vi "Impulse Response (V1.00).vi"(0 "wFormDSP Ref IN":refnum<class "GSwFormDSP.lvclass">, 5 "error in (no error)":errorcluster, 6 "ReInit All to Default?":bool, 7 "Application Name":string="GenUtil", 9 "State Queue":T1[](array[typedef])=["SC >>> Initialize"]) -> (19 "error out":errorcluster)   [LabVIEW 2020, in "SigMath.lvclass"]
uses:
  SigMath.lvclass
  API/Generic Utilities_class/utils/GenUtil State List.ctl
  API/GSwFormDSP_class/GSwFormDSP.lvclass
  <vilib>/Utility/sysdir.llb/System Directory Type.ctl
  API/GSwFormDSP_class/functions/Transfer Function Type.ctl
  C:/Users/fcharett/docsWork/coding/20openSourceSPWB/API/Generic Utilities_class/Generic Utilities.lvclass
  <vilib>/Platform/browser.llb/Open URL in Default Browser (path).vi
  <vilib>/addons/_AddQ/G#Object/G#Object.lvclass
  API/Generic Utilities_class/Generic Utilities.lvclass
  File IO/TEXT_class/TEXT.lvclass
panel:
  in  "Task":enum32{"Monitor", "Settings"}(tab)
  in  "Frequency Intervals [Hz]":u16(ring) items=["No Change", "0.10 Hz", "0.25 Hz", "0.50 Hz", "1.0 Hz", "2.0 Hz", "5.0 Hz", "10 Hz "]
  in  "Impulse Response":waveform(dbl)[](graph)
  out "Spectrum":cluster{dbl[], "Y":dbl[]}[](graph)
  in  "Exit":bool
  in  "Select CSV File":bool
  in  "AppData Folder":bool
  out "State History":string[](array[string])
  out "State Index":i32
  out "Exec Time":dbl
  out "Created New OBJ?":bool
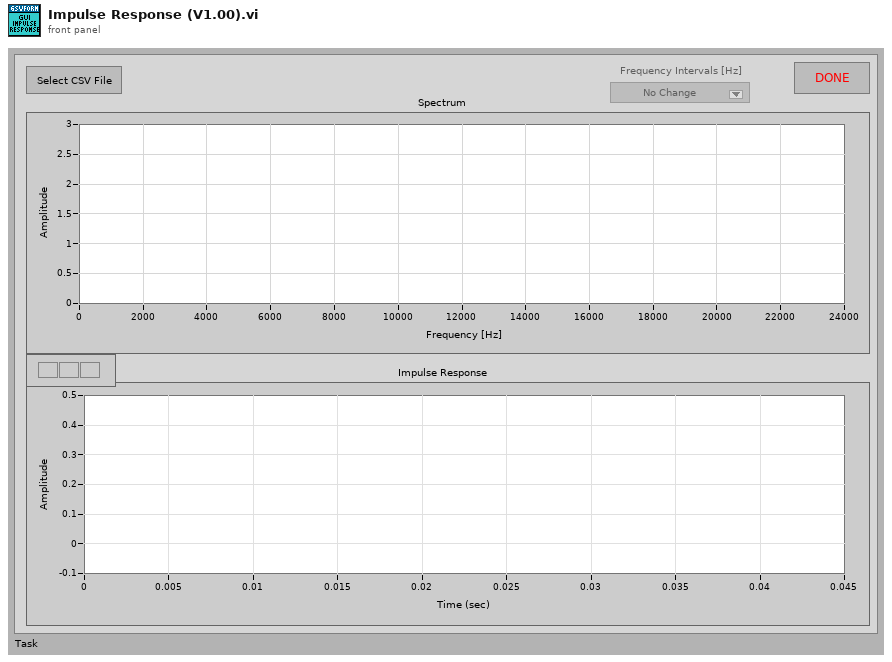
[diagram p1: front panel]
types:
  T1 = typedef "Generic Utilities.lvclass/GenUtil State List.ctl" = string
  T2 = typedef "GSwFormDSP.lvclass/Transfer Function Type.ctl" = enum16{"Magnitude", "Phase (Rad)", "Phase Unwrap (Rad)", "Phase (Degree)", "Phase Unwrap (Degree)", "Coherence"}
  T3 = enum32{"Invalid", "Standard", "Closed", "Hidden", "Minimized", "Maximized"}
  T4 = typedef "System Directory Type.ctl" = i32
  T5 = typedef "SigMath.lvclass/SigMath Data.ctl" = cluster{"New Time Data Obj?":bool, "GSwFormDSP":refnum<class "GSwFormDSP.lvclass">}
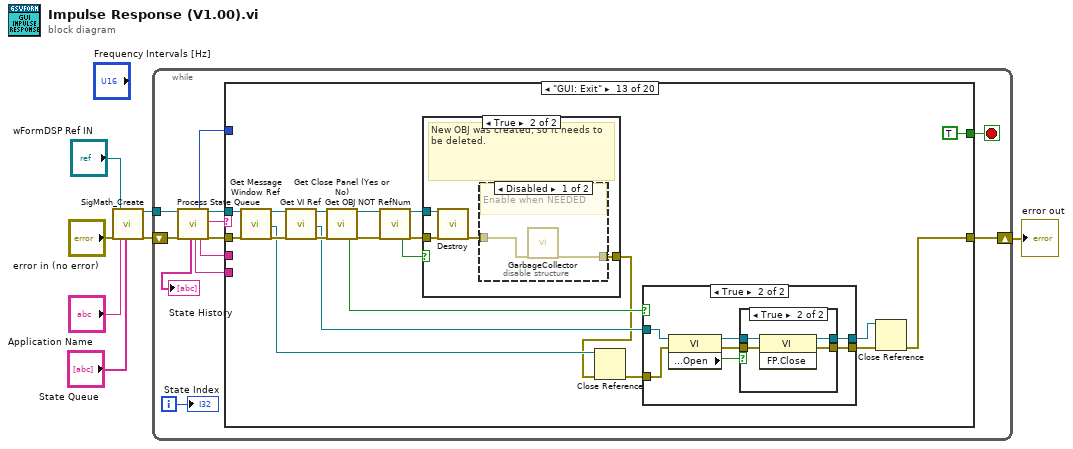
[diagram p0: block diagram]
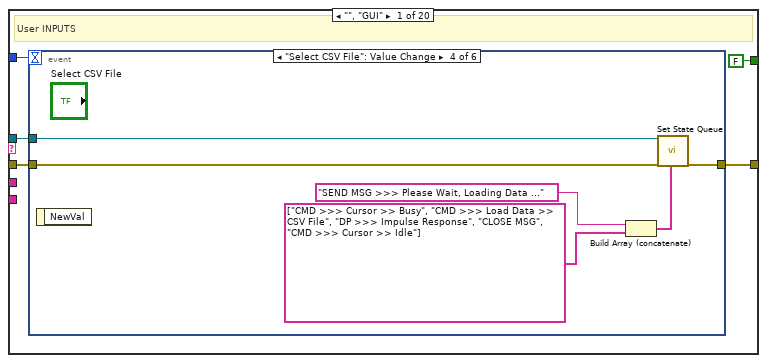
[diagram p2: hidden frame]
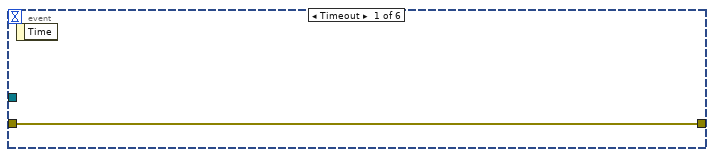
[diagram p3: hidden frame]
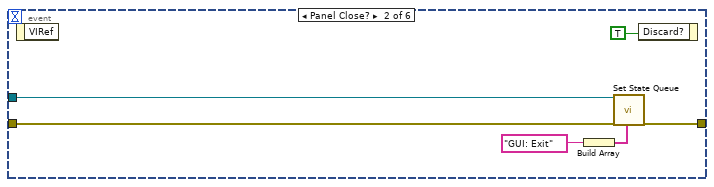
[diagram p4: hidden frame]
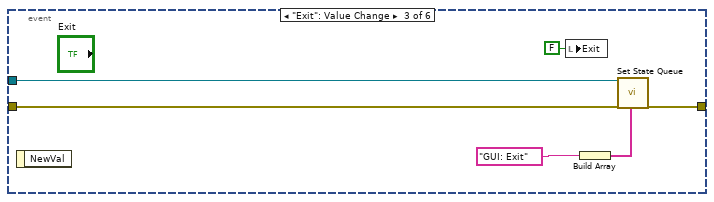
[diagram p5: hidden frame]
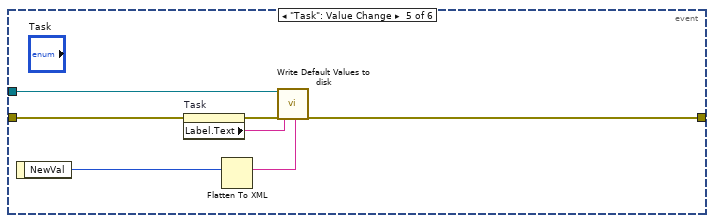
[diagram p6: hidden frame]
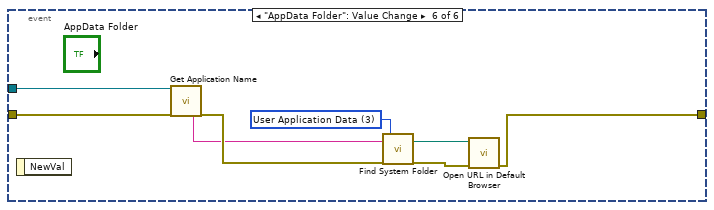
[diagram p7: hidden frame]
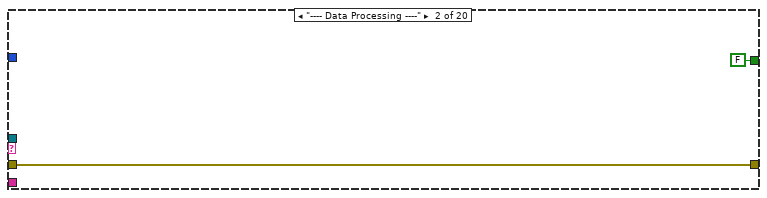
[diagram p8: hidden frame]
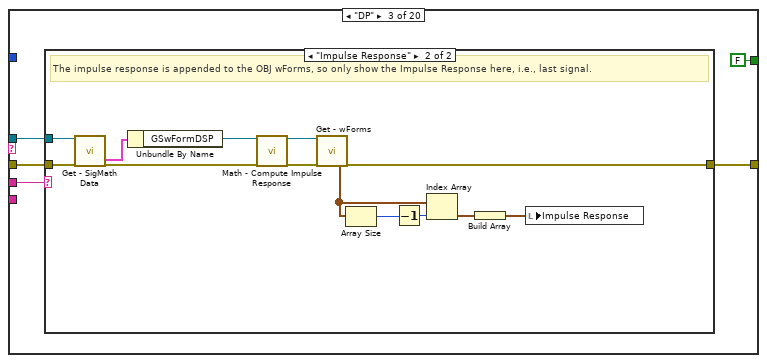
[diagram p9: hidden frame]
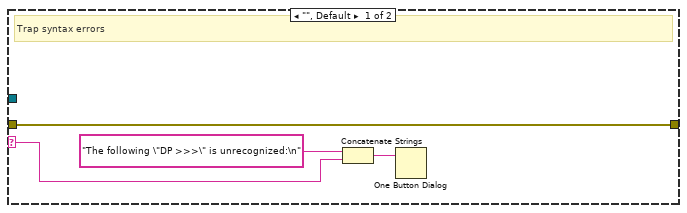
[diagram p10: hidden frame]
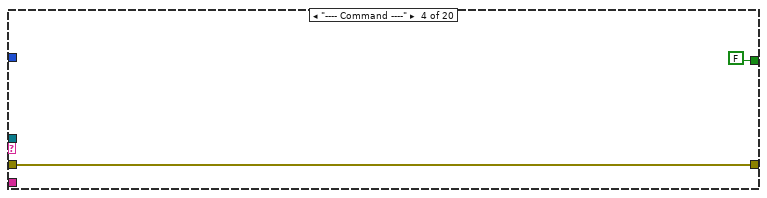
[diagram p11: hidden frame]
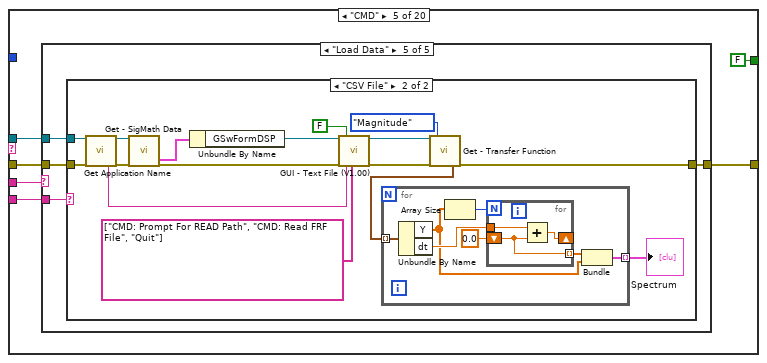
[diagram p12: hidden frame]
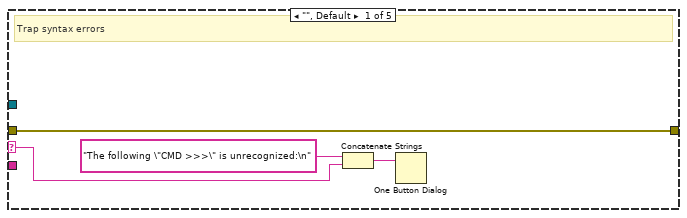
[diagram p13: hidden frame]
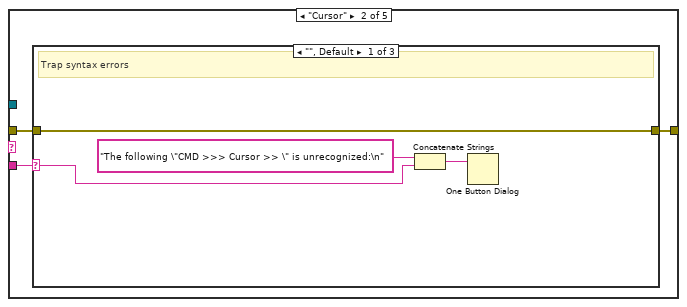
[diagram p14: hidden frame]
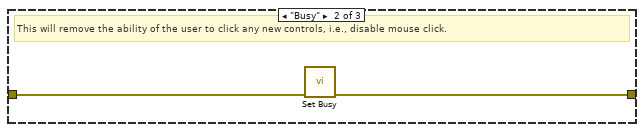
[diagram p15: hidden frame]
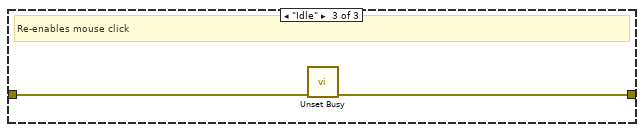
[diagram p16: hidden frame]
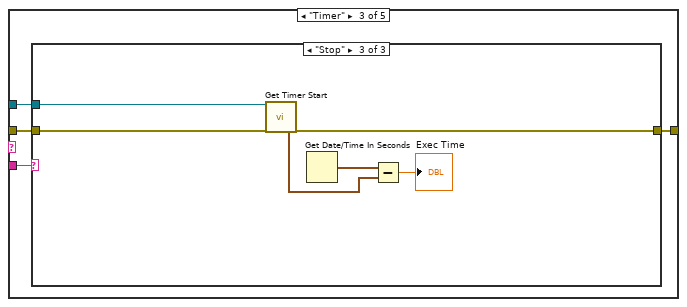
[diagram p17: hidden frame]
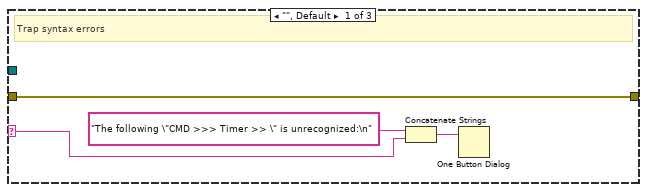
[diagram p18: hidden frame]
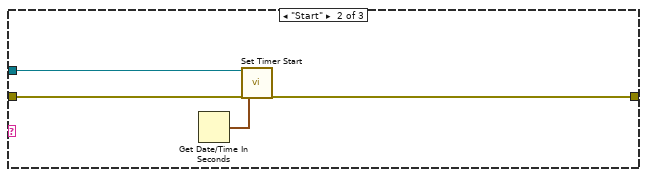
[diagram p19: hidden frame]
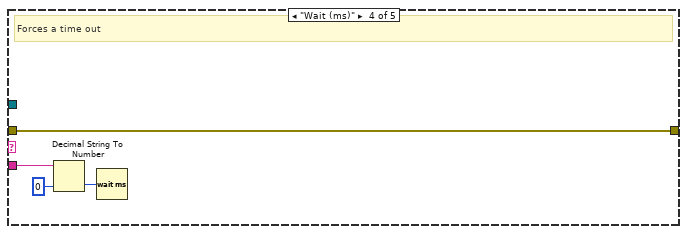
[diagram p20: hidden frame]
diagram:
  n1 = call "SigMath_Create.vi"("error in (no error)"="error in (no error)", "Time Data"="wFormDSP Ref IN", "Application Name"="Application Name", "State Queue"="State Queue") -> ("reference out"=w7:refnum<class "SigMath.lvclass">, "error out"=w6:errorcluster)  [unwired: 14 in]
  n2 = while {
    shift-right: [w11] -> w2
    shift-left: w6 -> [w16]
    tunnel: w7 -> [w17]
    i -> [w18]
    stop <- w19 stop-if-true
    n3 = call "Process State Queue.vi"("reference in"=w17, "error in (no error)"=w16) -> ("State History"=→"State History":string[], "Additional Options"=w8:string, "Timeout"=w15:i32, "State Option"=w10:string, "reference out"=w14:refnum<class "SigMath.lvclass">, "Current State"=w13:string, "error out"=w12:errorcluster)  [unwired: 10 in, 1 out]
    n4 = case shown="\"GUI: Exit\"" w13 {
      selector: w13 -> [_ _ _ _ _ _ _ _ _ _ _ _ _ _ _ _ w348 _ _ _]
      tunnel: w14 -> [w22 _ w61 _ w85 _ w169 _ w180 w214 _ w252 w271 w307 w332 _ _ _ _ w358]
      tunnel: [FALSE FALSE FALSE FALSE FALSE FALSE FALSE FALSE FALSE FALSE FALSE FALSE TRUE FALSE FALSE FALSE FALSE FALSE FALSE TRUE] -> w19
      tunnel: w15 -> [w23 _ _ _ _ _ _ _ _ _ _ _ _ _ _ _ _ _ _ _]
      tunnel: w10 -> [_ _ w64 _ w89 _ w165 _ w181 w211 _ _ _ w316 _ _ _ _ _ _]
      tunnel: w12 -> [w21 w59 w63 w83 w87 w162 w168 w176 w178 w213 w234 w249 w268 w306 w333 w344 w346 w351 w354 w357]
      tunnel: [w20 w59 w62 w83 w88 w162 w167 w176 w179 w212 w234 w241 w267 w304 w329 w344 w346 errorcluster {"status"=FALSE, "code"=0, "source"=""} ("error out") w354 w356] -> w11
      tunnel: w8 -> [_ _ _ _ w86 _ _ _ _ _ _ _ _ _ _ _ _ _ _ _]
      frame "", "GUI" {
        # "User INPUTS"
        n5 = event shown="[3] \"Select CSV File\": Value Change" {
          selector: _ -> [_ _ _ _ _ _]
          dyn-events: _ -> [_ _ _ _ _ _]
          timeout: w23 -> [_ _ _ _ _ _]
          tunnel: w22 -> [_ w30 w36 w42 w49 w57]
          tunnel: w21 -> [w25 w29 w34 w41 w46 w56]
          tunnel: [w25 w28 w35 w43 w44 w51] -> w20
          event Timeout {
            n6 = event-data() -> ()  [unwired: 1 in, 1 out]
          }
          event Panel Close? {
            n7 = event-data() -> ()  [unwired: 1 in, 1 out]
            n8 = Build Array(T1 "GUI: Exit" ("State List")) -> (w27:T1[])
            n9 = call "Set State Queue.vi"("reference in"=w30, "error in (no error)"=w29, "State Queue"=w27) -> ("error out"=w28:errorcluster)  [unwired: 15 in, 1 out]
            n10 = event-data("Discard?"=TRUE) -> ()  [unwired: 1 in, 1 out]
          }
          event "Exit": Value Change {
            n11 = event-data() -> ()  [unwired: 1 in, 1 out]
            n12 = local write "Exit"(FALSE ("Exit")) -> ()
            n13 = Build Array(T1 "GUI: Exit" ("State List")) -> (w33:T1[])
            n14 = call "Set State Queue.vi"("reference in"=w36, "error in (no error)"=w34, "State Queue"=w33) -> ("error out"=w35:errorcluster)  [unwired: 15 in, 1 out]
          }
          event "Select CSV File": Value Change {
            n15 = event-data() -> ()  [unwired: 1 in, 1 out]
            n16 = Build Array (concatenate)("SEND MSG >>> Please Wait, Loading Data ..." ("String"), T1[] ["CMD >>> Cursor >> Busy", "CMD >>> Load Data >> CSV File", "DP >>> Impulse Response", "CLOSE MSG", "CMD >>> Cursor >> Idle"] ("State Queue OUT")) -> (w38:T1[])
            n17 = call "Set State Queue.vi"("reference in"=w42, "error in (no error)"=w41, "State Queue"=w38) -> ("error out"=w43:errorcluster)  [unwired: 15 in, 1 out]
          }
          event "Task": Value Change {
            n18 = event-data() -> ("NewVal"=w50:enum32{"Monitor", "Settings"})  [unwired: 1 in]
            n19 = property on="Task" class="TabCtl (strict)"(error in=w46) -> (error out=w45:errorcluster, "Label.Text"=w48:string)  [unwired: 1 in, 1 out]
            n20 = Flatten To XML(6:w50) -> (2:w47:string)
            n21 = call-dynamic "Write Default Values to disk.vi"("reference in"=w49, "error in (no error)"=w45, "Control Label"=w48, "Value (XML String)"=w47) -> ("error out"=w44:errorcluster)  [unwired: 14 in, 1 out]
          }
          event "AppData Folder": Value Change {
            w58 = T4 3 items=["User Home"=0, "User Desktop"=1, "User Documents"=2, "User Application Data"=3, "User Preferences"=4, "User Temporary"=5, "Public Documents"=6, "Public Application Data"=7, "Public Preferences"=8, "Public Cache"=13, "System Core Libraries"=9, "System Installed Libraries"=10, "Application Files"=11, "Boot Volume Root"=12] ("system directory type")
            n22 = event-data() -> ()  [unwired: 1 in, 1 out]
            n23 = call "Get Application Name.vi"("reference in"=w57, "error in (no error)"=w56) -> ("Application Name"=w54:string, "error out"=w55:errorcluster)  [unwired: 15 in, 1 out]
            n24 = call "Find System Folder.vi"("Application Name"=w54, "error in (no error)"=w55, "system directory type"=w58) -> ("System Folder"=w53:path, "error out"=w52:errorcluster)  [unwired: 15 in]
            n25 = call-poly <vilib>:"Open URL in Default Browser.vi"("error in (no error)"=w52, "path"=w53) -> ("error out"=w51:errorcluster)  [unwired: 4 in, 1 out]
          }
        }
      }
      frame "---- Data Processing ----" {
      }
      frame "DP" {
        n26 = case shown="\"Impulse Response\"" w64 {
          selector: w64 -> [w67 _]
          tunnel: [w66 w80] -> w62
          tunnel: w63 -> [w66 w74]
          tunnel: w61 -> [_ w73]
          frame "", Default {
            # "Trap syntax errors"
            n27 = Concatenate Strings("The following \"DP >>>\" is unrecognized:\n", w67) -> (w68:string)
            n28 = One Button Dialog(message=w68) -> ()  [unwired: 1 in, 1 out]
          }
          frame "Impulse Response" {
            # "The impulse response is appended to the OBJ wForms, so only show the Impulse Response here, i.e., last signal."
            n29 = call "Get - SigMath Data.vi"("reference in"=w73, "error in (no error)"=w74) -> ("SigMath Data"=w72:T5, "error out"=w71:errorcluster)  [unwired: 15 in, 1 out]
            n30 = Unbundle By Name(w72) -> ("GSwFormDSP"=w70:refnum<class "GSwFormDSP.lvclass">)
            n31 = call "Math - Compute Impulse Response.vi"("reference in"=w70, "error in (no error)"=w71) -> ("reference out"=w82:refnum<class "GSwFormDSP.lvclass">, "error out"=w81:errorcluster)  [unwired: 16 in]
            n32 = call-dynamic "Get - wForms.vi"("reference in"=w82, "error in (no error)"=w81) -> ("wForms"=w79:waveform(dbl)[], "error out"=w80:errorcluster)  [unwired: 14 in, 2 out]
            n33 = Array Size(array=w79) -> (size(s)=w78:i32)
            n34 = Decrement(x=w78) -> (x-1=w75:i32)
            n35 = Index Array(array=w79, index=w75) -> (element=w76:waveform(dbl))
            n36 = Build Array(w76) -> (w77:waveform(dbl)[])
            n37 = local write "Impulse Response"(w77) -> ()
          }
        }
      }
      frame "---- Command ----" {
      }
      frame "CMD" {
        n38 = case shown="\"Load Data\"" w89 {
          selector: w89 -> [w92 _ _ _ _]
          tunnel: [w91 w96 w108 w127 w129] -> w88
          tunnel: w87 -> [w91 w95 w107 w127 w130]
          tunnel: w86 -> [_ w97 w109 w124 w131]
          tunnel: w85 -> [_ _ w106 _ w128]
          frame "", Default {
            # "Trap syntax errors"
            n39 = Concatenate Strings("The following \"CMD >>>\" is unrecognized:\n", w92) -> (w93:string)
            n40 = One Button Dialog(message=w93) -> ()  [unwired: 1 in, 1 out]
          }
          frame "Cursor" {
            n41 = case shown="\"\", Default" w97 {
              selector: w97 -> [w99 _ _]
              tunnel: [w98 w102 w104] -> w96
              tunnel: w95 -> [w98 w103 w105]
              frame "", Default {
                # "Trap syntax errors"
                n42 = Concatenate Strings("The following \"CMD >>> Cursor >> \" is unrecognized:\n", w99) -> (w100:string)
                n43 = One Button Dialog(message=w100) -> ()  [unwired: 1 in, 1 out]
              }
              frame "Busy" {
                # "This will remove the ability of the user to click any new controls, i.e., disable mouse click."
                n44 = call <vilib>:"Set Busy.vi"("error in (no error)"=w103) -> ("error out"=w102:errorcluster)  [unwired: 9 in, 1 out]
              }
              frame "Idle" {
                # "Re-enables mouse click"
                n45 = call <vilib>:"Unset Busy.vi"("error in (no error)"=w105) -> ("error out"=w104:errorcluster)  [unwired: 10 in]
              }
            }
          }
          frame "Timer" {
            n46 = case shown="\"Stop\"" w109 {
              selector: w109 -> [w111 _ _]
              tunnel: [w110 w115 w120] -> w108
              tunnel: w107 -> [w110 w116 w121]
              tunnel: w106 -> [_ w117 w122]
              frame "", Default {
                # "Trap syntax errors"
                n47 = Concatenate Strings("The following \"CMD >>> Timer >> \" is unrecognized:\n", w111) -> (w112:string)
                n48 = One Button Dialog(message=w112) -> ()  [unwired: 1 in, 1 out]
              }
              frame "Start" {
                n49 = Get Date/Time In Seconds() -> (seconds since 1Jan1904=w114:timestamp)
                n50 = call "Set Timer Start.vi"("reference in"=w117, "error in (no error)"=w116, "Timer Start"=w114) -> ("error out"=w115:errorcluster)  [unwired: 15 in, 1 out]
              }
              frame "Stop" {
                n51 = call "Get Timer Start.vi"("reference in"=w122, "error in (no error)"=w121) -> ("Timer Start"=w119:timestamp, "error out"=w120:errorcluster)  [unwired: 15 in, 1 out]
                n52 = Get Date/Time In Seconds() -> (seconds since 1Jan1904=w123:timestamp)
                n53 = Subtract(x=w123, y=w119) -> (x-y=→"Exec Time":dbl)
              }
            }
          }
          frame "Wait (ms)" {
            # "Forces a time out"
            n54 = Decimal String To Number(string=w124, default (0L)=u32 0 ("default (0 I32)")) -> (number=w125:u32)  [unwired: 1 in, 1 out]
            n55 = Wait (ms)(milliseconds to wait=w125) -> ()  [unwired: 1 out]
          }
          frame "Load Data" {
            n56 = case shown="\"CSV File\"" w131 {
              selector: w131 -> [w132 _]
              tunnel: w130 -> [w133 w150]
              tunnel: [w133 w143] -> w129
              tunnel: w128 -> [_ w151]
              frame "", Default {
                n57 = Concatenate Strings("The following \"CMD >>> Load Data >> \" is unrecognized:\n", w132) -> (w134:string)
                n58 = One Button Dialog(message=w134) -> ()  [unwired: 1 in, 1 out]
              }
              frame "CSV File" {
                n59 = call "Get Application Name.vi"("reference in"=w151, "error in (no error)"=w150) -> ("Application Name"=w149:string, "reference out"=w139:refnum<class "SigMath.lvclass">, "error out"=w138:errorcluster)  [unwired: 15 in]
                n60 = call "Get - SigMath Data.vi"("reference in"=w139, "error in (no error)"=w138) -> ("SigMath Data"=w140:T5, "error out"=w137:errorcluster)  [unwired: 15 in, 1 out]
                n61 = Unbundle By Name(w140) -> ("GSwFormDSP"=w136:refnum<class "GSwFormDSP.lvclass">)
                n62 = call "GUI - Text File (V1.00).vi"("Time Data IN"=w136, "error in (no error)"=w137, "Inlude Time Vector"=FALSE, "Application Name"=w149, "State Queue"=string[] ["CMD: Prompt For READ Path", "CMD: Read FRF File", "Quit"]) -> ("Time Data DUP"=w146:refnum<class "GSwFormDSP.lvclass">, "error out"=w144:errorcluster)  [unwired: 13 in]
                n63 = call "Get - Transfer Function.vi"("reference in"=w146, "error in (no error)"=w144, "Transfer Function Type"=Transfer_Function_Type."Magnitude") -> ("Data"=w142:waveform(dbl)[], "error out"=w143:errorcluster)  [unwired: 13 in, 2 out]
                n64 = for {
                  tunnel: w142 -> [w158] mode=indexing
                  tunnel: [w152] -> w141 mode=indexing
                  n65 = Unbundle By Name(w158) -> ("Y"=w153:dbl[], "dt"=w156:dbl)
                  n66 = Array Size(array=w153) -> (size(s)=w157:i32)
                  n67 = for {
                    N: w157 -> [_]
                    shift-right: [w160] -> _
                    shift-left: 0.0 -> [w159]
                    tunnel: w156 -> [w161]
                    tunnel: [w159] -> w154 mode=indexing
                    n68 = Add(x=w161, y=w159) -> (x+y=w160:dbl)
                  }
                  n69 = Bundle(w154, "Y"=w153) -> (w152:cluster{dbl[], "Y":dbl[]})  [unwired: 1 in]
                }
                "Spectrum" <- w141
              }
            }
          }
        }
      }
      frame "---- Scripts ----" {
      }
      frame "SC" {
        n70 = case shown="\"Initialize\"" w165 {
          selector: w165 -> [w172 _]
          tunnel: [string[] [] ("State Queue OUT") string[] ["GUI: Initialize Ref", "CTRL >>> Task Tab", "FP >>> Open"] ("State Queue OUT")] -> w166
          frame "False", Default {
            n71 = Concatenate Strings("The following \"Script\" is unrecognized:\n", w172) -> (w173:string)
            n72 = One Button Dialog(message=w173) -> ()  [unwired: 1 in, 1 out]
          }
          frame "Initialize" {
          }
        }
        n73 = call "Set State Queue.vi"("reference in"=w169, "error in (no error)"=w168, "State Queue Options"=enum16{"Replace", "Append", "Prepend"}."Prepend", "State Queue"=w166) -> ("error out"=w167:errorcluster)  [unwired: 14 in, 1 out]
      }
      frame "---- Front Panel Mgmt ----" {
      }
      frame "CTRL" {
        n74 = case shown="\"unknown\", Default" w181 {
          selector: w181 -> [w185 _]
          tunnel: w180 -> [_ w189]
          tunnel: [w183 w187] -> w179
          tunnel: w178 -> [w183 w188]
          frame "unknown", Default {
            n75 = Concatenate Strings("The following control name is unrecognized:\n", w185) -> (w184:string)
            n76 = One Button Dialog(message=w184) -> ()  [unwired: 1 in, 1 out]
          }
          frame "Task Tab" {
            n77 = disable-structure shown="Enabled" {
              disable-tunnel: [w200 0] -> w191
              disable-tunnel: [w198 w210] -> w190
              disable-tunnel: w189 -> [w197 _]
              disable-tunnel: w188 -> [w195 w210]
              frame Disabled {
                n78 = property on="Task" class="TabCtl (strict)"(error in=w195) -> (error out=w196:errorcluster, "Label.Text"=w194:string, "Value"=w199:enum32{"Monitor", "Settings"})  [unwired: 1 in, 1 out]
                n79 = call-dynamic "Read Default Values from Disk.vi"("reference in"=w197, "error in (no error)"=w196, "Control Label"=w194) -> (17:w193, "error out"=w192:errorcluster)  [unwired: 13 in, 2 out]
                n80 = case shown="\"\"" w193 {
                  selector: w193 -> [w206 _]
                  tunnel: [w201 w208] -> w200
                  tunnel: w199 -> [w203 w208]
                  tunnel: w192 -> [w204 w207]
                  tunnel: [w204 w207] -> w198
                  frame "anything", Default {
                    n81 = Unflatten From XML(xml string=w206, type=w203, error in (no error)=w204) -> (value=w202:enum32{"Monitor", "Settings"}, error out=w205:errorcluster)
                    n82 = Select(t=w203, s=w205, f=w202) -> (s? t:f=w201:enum32{"Monitor", "Settings"})
                  }
                  frame "" {
                    # "Either the file was not found or there was some error"
                  }
                }
              }
              frame Enabled {
              }
            }
            n83 = property on="Task" class="TabCtl (strict)"(error in=w190, "Value"=w191) -> (error out=w187:errorcluster)  [unwired: 1 in, 1 out]
          }
        }
      }
      frame "FP" {
        n84 = case shown="\"Open\"" w211 {
          selector: w211 -> [w216 _]
          tunnel: w214 -> [_ w224]
          tunnel: w213 -> [w217 w223]
          tunnel: [w217 w220] -> w212
          frame "unknown", Default {
            n85 = Concatenate Strings("The following FP Command name is unrecognized:\n", w216) -> (w218:string)
            n86 = One Button Dialog(message=w218) -> ()  [unwired: 1 in, 1 out]
          }
          frame "Open" {
            n87 = call-dynamic "Get VI Ref.vi"("reference in"=w224, "error in (no error)"=w223) -> ("GUI VI Ref"=w221:refnum<vi>, "error out"=w222:errorcluster)  [unwired: 14 in, 2 out]
            n88 = property class="VI"(reference=w221, error in=w222) -> (reference out=w226:refnum<vi>, error out=w227:errorcluster, "Front Panel.Open"=w225:bool)
            n89 = case shown="False" w225 {
              tunnel: [w230 w233] -> w220
              tunnel: w227 -> [w229 w233]
              tunnel: w226 -> [w228 _]
              frame False {
                n90 = invoke class="VI" method="FP.Open"(reference=w228, error in=w229, "Activate"=TRUE, "State"=T3."Standard") -> (error out=w230:errorcluster)  [unwired: 1 in, 4 out]
              }
              frame True {
              }
            }
          }
        }
      }
      frame "---- GUI Functions ----" {
      }
      frame "GUI: Initialize Ref" {
        n91 = control-ref of="GUI Reference"() -> (w248:refnum<vi>)
        n92 = call "Set VI Ref.vi"("reference in"=w252, "error in (no error)"=w249, "ReInit All to Default?"="ReInit All to Default?", "GUI VI Ref"=w248) -> ("reference out"=w251:refnum<class "SigMath.lvclass">, "error out"=w247:errorcluster)  [unwired: 14 in]
        n93 = call "Set Close Panel (Yes or No).vi"("reference in"=w251, "error in (no error)"=w247) -> ("reference out"=w250:refnum<class "SigMath.lvclass">, "error out"=w246:errorcluster)  [unwired: 16 in]
        n94 = call "Set Message Window Ref.vi"("reference in"=w250, "error in (no error)"=w246) -> ("reference out"=w243:refnum<class "SigMath.lvclass">, "error out"=w244:errorcluster)  [unwired: 16 in]
        n95 = call "Get - SigMath Data.vi"("reference in"=w243, "error in (no error)"=w244) -> ("SigMath Data"=w238:T5, "error out"=w242:errorcluster)  [unwired: 15 in, 1 out]
        n96 = Unbundle By Name(w238) -> ("GSwFormDSP"=w236:refnum<class "GSwFormDSP.lvclass">, "New Time Data Obj?"=w237:bool)
        "Created New OBJ?" <- w237
        n97 = case shown="True" w237 {
          tunnel: w242 -> [w254 w258]
          tunnel: [w254 w256] -> w241
          tunnel: w236 -> [_ w255]
          frame False {
          }
          frame True {
            # "Created a new OBJ, so need to initialize the wForm ref"
            n98 = call "Set - wForms.vi"("reference in"=w255, "error in (no error)"=w258, "Init wForms"=TRUE, "wForms"="Impulse Response") -> ("error out"=w256:errorcluster)  [unwired: 14 in, 1 out]
          }
        }
        n99 = local write "Impulse Response"(waveform(dbl)[] [] ("Impulse Response")) -> ()
        n100 = local write "Spectrum"(cluster{dbl[], "Y":dbl[]}[] [{[], "Y"=[]}] ("Spectrum")) -> ()
      }
      frame "GUI: Exit" {
        n101 = call-dynamic "Get Message Window Ref.vi"("reference in"=w271, "error in (no error)"=w268) -> ("reference out"=w270:refnum<class "SigMath.lvclass">, "Msg Win Ref"=w266:refnum<vi>, "error out"=w269:errorcluster)  [unwired: 15 in]
        n102 = call-dynamic "Get VI Ref.vi"("reference in"=w270, "error in (no error)"=w269) -> ("reference out"=w274:refnum<class "SigMath.lvclass">, "GUI VI Ref"=w272:refnum<vi>, "error out"=w273:errorcluster)  [unwired: 14 in, 1 out]
        n103 = call-dynamic "Get Close Panel (Yes or No).vi"("reference in"=w274, "error in (no error)"=w273) -> ("Close Panel?"=w275:bool, "reference out"=w264:refnum<class "SigMath.lvclass">, "error out"=w265:errorcluster)  [unwired: 15 in]
        n104 = call-dynamic "Get OBJ NOT RefNum.vi"("reference in"=w264, "error in (no error)"=w265) -> ("OBJ not a refnum?"=w263:bool, "reference out"=w262:refnum<class "SigMath.lvclass">, "error out"=w261:errorcluster)  [unwired: 15 in]
        n105 = case shown="True" w263 {
          tunnel: [w280 w283] -> w260
          tunnel: w262 -> [_ w282]
          tunnel: w261 -> [w280 w281]
          frame False {
            # "The OBJ already exist, indicating this is a dialog box or sub-vi so do NOT destroy the original OBJ."
          }
          frame True {
            # "New OBJ was created, so it needs to be deleted."
            n106 = call-dynamic "Destroy.vi"("reference in"=w282, "error in (no error)"=w281) -> ("error out"=w284:errorcluster)  [unwired: 16 in, 1 out]
            n107 = disable-structure shown="Disabled" {
              disable-tunnel: w284 -> [w286 w287]
              disable-tunnel: [w285 w287] -> w283
              frame Disabled {
                # "Enable when NEEDED"
                n108 = call <vilib>:"GarbageCollector.vi"("error in (no error)"=w286) -> ("error out"=w285:errorcluster)  [unwired: 16 in, 2 out]
              }
              frame Enabled {
              }
            }
          }
        }
        n109 = Close Reference(reference=w266, error in (no error)=w260) -> (error out=w278:errorcluster)
        n110 = case shown="True" w275 {
          tunnel: w278 -> [w289 w293]
          tunnel: [w289 w292] -> w276
          tunnel: [w288 w291] -> w277
          tunnel: w272 -> [w288 w290]
          frame False {
          }
          frame True {
            n111 = property class="VI"(reference=w290, error in=w293) -> (reference out=w295:refnum<vi>, error out=w294:errorcluster, "Front Panel.Open"=w296:bool)
            n112 = case shown="True" w296 {
              tunnel: [w298 w302] -> w292
              tunnel: w294 -> [w298 w301]
              tunnel: w295 -> [w297 w300]
              tunnel: [w297 w299] -> w291
              frame False {
              }
              frame True {
                n113 = invoke class="VI" method="FP.Close"(reference=w300, error in=w301) -> (reference out=w299:refnum<vi>, error out=w302:errorcluster)  [unwired: 1 in, 1 out]
              }
            }
          }
        }
        n114 = Close Reference(reference=w277, error in (no error)=w276) -> (error out=w267:errorcluster)
      }
      frame "SEND MSG" {
        n115 = call-dynamic "Get Message Window Ref.vi"("reference in"=w307, "error in (no error)"=w306) -> ("Msg Win Ref"=w303:refnum<vi>, "error out"=w305:errorcluster)  [unwired: 15 in, 1 out]
        n116 = property class="VI"(reference=w303, error in=w305) -> (reference out=w309:refnum<vi>, error out=w308:errorcluster, "Front Panel.Open"=w310:bool)
        n117 = case shown="False" w310 {
          tunnel: [w324 w328] -> w312
          tunnel: w308 -> [w319 w328]
          tunnel: w309 -> [w321 w327]
          tunnel: [w323 w327] -> w311
          frame False {
            w322 = FALSE ("Wait Until Done")
            n118 = invoke class="VI" method="Run VI"(reference=w321, error in=w319, "Wait until done"=w322, "Auto Dispose Ref"=w322) -> (reference out=w320:refnum<vi>, error out=w318:errorcluster)  [unwired: 1 in, 3 out]
            n119 = invoke class="VI" method="FP.Open"(reference=w320, error in=w318, "Activate"=TRUE, "State"=T3."Standard") -> (reference out=w323:refnum<vi>, error out=w324:errorcluster)  [unwired: 1 in, 3 out]
          }
          frame True {
          }
        }
        n120 = Concatenate Strings("\r\n", w316) -> (w315:string)
        n121 = invoke class="VI" method="Ctrl Val.Set"(reference=w311, error in=w312, "Control Name"="Message", "Value"=w315) -> (error out=w304:errorcluster)  [unwired: 1 in, 4 out]
      }
      frame "CLOSE MSG" {
        n122 = call-dynamic "Get Message Window Ref.vi"("reference in"=w332, "error in (no error)"=w333) -> ("Msg Win Ref"=w330:refnum<vi>, "error out"=w331:errorcluster)  [unwired: 15 in, 1 out]
        n123 = property class="VI"(reference=w330, error in=w331) -> (reference out=w335:refnum<vi>, error out=w336:errorcluster, "Front Panel.Open"=w334:bool)
        n124 = case shown="True" w334 {
          tunnel: [w338 w339] -> w329
          tunnel: w336 -> [w338 w343]
          tunnel: w335 -> [_ w342]
          frame False {
          }
          frame True {
            n125 = invoke class="VI" method="FP.Close"(reference=w342, error in=w343) -> (reference out=w341:refnum<vi>, error out=w340:errorcluster)  [unwired: 1 in, 1 out]
            n126 = invoke class="VI" method="Abort VI"(reference=w341, error in=w340) -> (error out=w339:errorcluster)  [unwired: 1 in, 2 out]
          }
        }
      }
      frame "---- Miscelleneous ----" {
      }
      frame "unknown", Default {
        n127 = Concatenate Strings("The following state is unrecognized?\n", w348) -> (w347:string)
        n128 = One Button Dialog(message=w347) -> ()  [unwired: 1 in, 1 out]
      }
      frame "Error" {
        n129 = call <vilib>:"General Error Handler.vi"("error in (no error)"=w351) -> ()  [unwired: 10 in, 5 out]
      }
      frame "Next" {
        # "This is an empty case used so the queue does NOT stop if there is an empty string between two valid states!"
      }
      frame "Quit" {
        # "WARNING!, If the state machine crash, then it will also \"Quit\"??"
        # "This is the case used to simply exit when this GUI is used as a SubVI!"
        n130 = call-dynamic "Destroy.vi"("reference in"=w358, "error in (no error)"=w357) -> ("error out"=w356:errorcluster)  [unwired: 16 in, 1 out]
      }
    }
    "State Index" <- w18
  }
  "error out" <- w2
